vi "ActionVIOnCompile.vi"(8 "error in (no error)":errorcluster, 11 "Device Item Ref in":T1 format="%.0x") -> (0 "error out":errorcluster)   [LabVIEW 2012, in "PXImc System Explorer.lvlib"]
uses:
  PXImc System Explorer.lvlib
  <vilib>/NI Veristand/Custom Device API/Custom Device Item Ref.ctl
  Shared/Compiled Data.ctl
  Shared/Constants.vi
  <vilib>/NI Veristand/Custom Device API/Get Item Property (String).vi
  <vilib>/NI Veristand/Custom Device API/Get Item Property (U16).vi
  <vilib>/NI Veristand/Custom Device API/Set Item Property (Variant).vi
  Shared/PXImc Shared.lvlib
  <vilib>/NI Veristand/Custom Device API/Custom Device API.lvlib
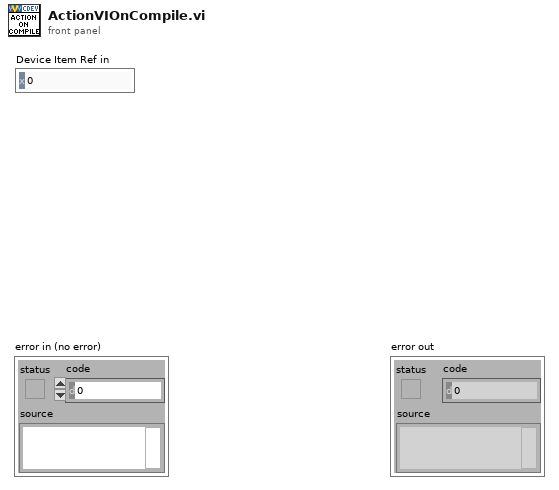
[diagram p1: front panel]
types:
  T1 = typedef "Custom Device API.lvlib/Custom Device Item Ref.ctl" = u64
  T2 = typedef "PXImc Shared.lvlib/Compiled Data.ctl" = cluster{"My write ID":u16, "Remote write ID":u16, "Module Name":string, "Name":string}
  T3 = typedef "Custom Device API.lvlib/Custom Device Item Info.ctl" = cluster{"Name":string, "Is Channel":bool, "GUID":string, "Is Waveform":bool}
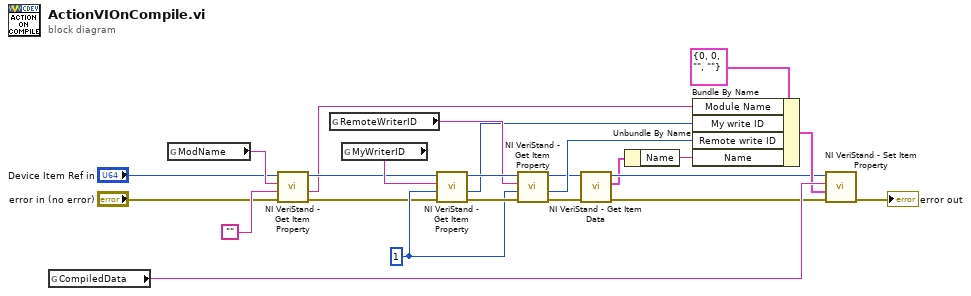
[diagram p0: block diagram]
diagram:
  w16 = u16 1 ("Default Value")
  n1 = global read "Constants.vi" "CompiledData"() -> (w22:string)
  n2 = global read "Constants.vi" "ModName"() -> (w13:string)
  n3 = call-poly <vilib>:"NI VeriStand - Get Item Property.vi"("error in (no error)"="error in (no error)", "Default Value"="", "Property Name"=w13, "Item Ref in"="Device Item Ref in") -> ("error out"=w15:errorcluster, "Value"=w9:string, "Item Ref out"=w14:T1)  [unwired: 4 in, 1 out]
  n4 = global read "Constants.vi" "RemoteWriterID"() -> (w17:string)
  n5 = global read "Constants.vi" "MyWriterID"() -> (w19:string)
  n6 = call-poly <vilib>:"NI VeriStand - Get Item Property.vi"("error in (no error)"=w15, "Default Value"=w16, "Property Name"=w19, "Item Ref in"=w14) -> ("error out"=w20:errorcluster, "Value"=w8:u16, "Item Ref out"=w18:T1)  [unwired: 4 in, 1 out]
  n7 = call-poly <vilib>:"NI VeriStand - Get Item Property.vi"("error in (no error)"=w20, "Default Value"=w16, "Property Name"=w17, "Item Ref in"=w18) -> ("error out"=w7:errorcluster, "Value"=w6:u16, "Item Ref out"=w4:T1)  [unwired: 4 in, 1 out]
  n8 = call <vilib>:"NI VeriStand - Get Item Data.vi"("error in (no error)"=w7, "Item Ref in"=w4) -> ("error out"=w5:errorcluster, "Item Info"=w2:T3, "Item Ref out"=w3:T1)  [unwired: 6 in, 1 out]
  n9 = Unbundle By Name(w2) -> ("Name"=w1:string)
  n10 = Bundle By Name(cluster=T2 {"My write ID"=0, "Remote write ID"=0, "Module Name"="", "Name"=""} ("Compiled Data"), "Module Name"=w9, "My write ID"=w8, "Remote write ID"=w6, "Name"=w1) -> (w21:T2)
  n11 = call-poly <vilib>:"NI VeriStand - Set Item Property.vi"("error in (no error)"=w5, "Value"=w21, "Property Name"=w22, "Item Ref in"=w3) -> ("error out"=→"error out":errorcluster)  [unwired: 5 in, 2 out]
